vi "Loop Period.vi"(8 "error in (no error)":errorcluster, 11 "PID in":refnum<class "PID.lvclass">) -> (0 "error out":errorcluster, 3 "PID out":refnum<class "PID.lvclass">)   [LabVIEW 2025, in "PID.lvlib" / "PID.lvclass"]
uses:
  PID.lvclass
  PID.lvclass/PID.ctl
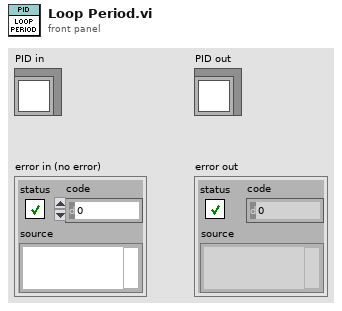
[diagram p1: front panel]
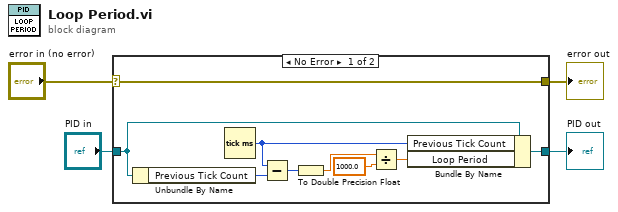
[diagram p0: block diagram]
diagram:
  n1 = case shown="No Error" "error in (no error)" {
    selector: "error in (no error)" -> [w13 w15]
    tunnel: [w13 w15] -> w3
    tunnel: [w5 w14] -> w1
    tunnel: "PID in" -> [w11 w14]
    frame No Error {
      n2 = Unbundle By Name(w11) -> ("Previous Tick Count"=w12:u32)
      n3 = Tick Count (ms)() -> (millisecond timer value=w10:u32)
      n4 = Subtract(x=w10, y=w12) -> (x-y=w9:u32)
      n5 = To Double Precision Float(number=w9) -> (double precision float=w6:dbl)
      n6 = Divide(x=w6, y=1000.0) -> (x/y=w7:dbl)
      n7 = Bundle By Name(cluster=w11, "Previous Tick Count"=w10, "Loop Period"=w7) -> (w5:refnum<class "PID.lvclass">)
    }
    frame Error {
    }
  }
  "error out" <- w3
  "PID out" <- w1
